vi "KeyAdd.vi"(8 "error in (no error)":errorcluster caption="错误输入（无错误）", 10 "键名":string, 11 "段名":string) -> (0 "error out":errorcluster caption="错误输出")   [LabVIEW 2020]
uses:
  <vilib>/Utility/config.llb/Write Key (Boolean).vi
  <vilib>/Utility/config.llb/NI_LVConfig.lvlib
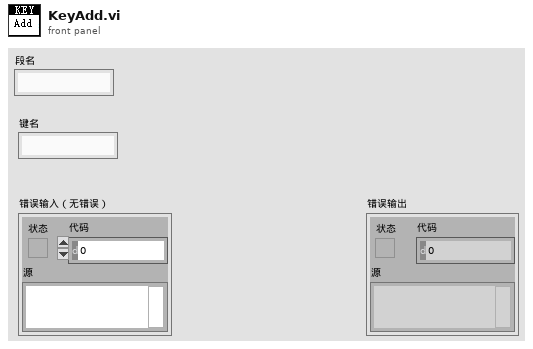
[diagram p1: front panel]
types:
  T1 = typedef "NI_LVConfig.lvlib/Config Data RefNum.ctl" = refnum<k1>
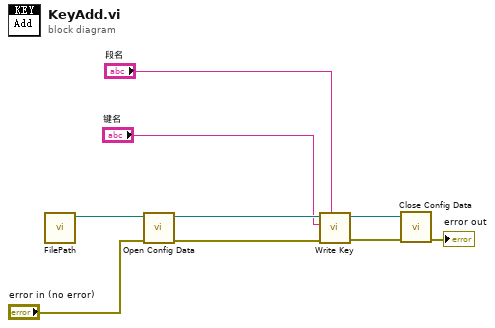
[diagram p0: block diagram]
diagram:
  n1 = call "FilePath.vi"() -> ("添加的路径"=w3:path)  [unwired: 11 in]
  n2 = call <vilib>:"Open Config Data.vi"("error in (no error)"="error in (no error)", "configuration file path"=w3) -> ("error out"=w6:errorcluster, "refnum"=w9:T1)  [unwired: 7 in, 1 out]
  n3 = call-poly <vilib>:"Write Key.vi"("section"="段名", "error in (no error)"=w6, "key"="键名", "refnum"=w9) -> ("error out"=w4:errorcluster, "refnum out"=w5:T1)  [unwired: 5 in, 1 out]
  n4 = call <vilib>:"Close Config Data.vi"("error in (no error)"=w4, "refnum"=w5) -> ("error out"=→"error out":errorcluster)  [unwired: 8 in, 1 out]
